vi "Passing Data to a .NET Event Callback.vi"() -> ()   [LabVIEW 2023]
doc: "This vi demonstrates how to use the .NET event callback to fire an event on a value change. This example uses a C# project file to create the event. The constructor from this project is then used to register the event."
uses:
  c:/dev/_r/4/eng/lv-core/lvpostprocessingd/lv_mc_x86_64/dist_i386/examples/Connectivity/Dot NET/EventExample.dll
  EventExample.dll
panel:
  in  "Knob":dbl(knob) scale=0.0..10.0
  in  "Stop":bool
  out "Meter":dbl(knob) scale=0.0..10.0
  # "Overview: Demonstrates how to configure a .NET Event Callback, then pass data to the callback VI when a Value Changed event fires.\nRequirements: Windows\nInstructions:\n1. Run the VI.\n2. Change the Knob value. The value of Meter will be updated based on the knob value sent to the .NET Event Callback VI.\n3. Click Stop to stop the VI."
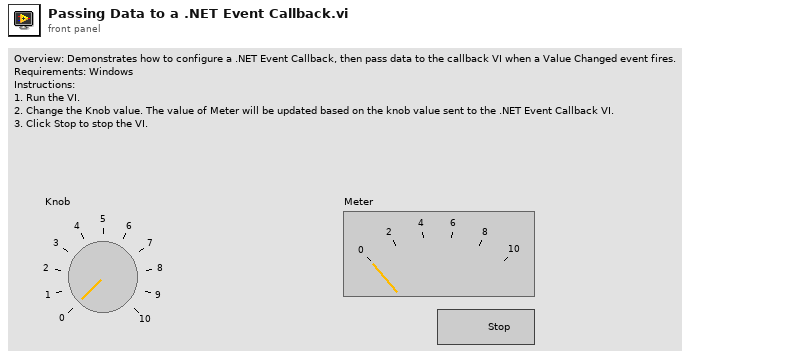
[diagram p1: front panel]
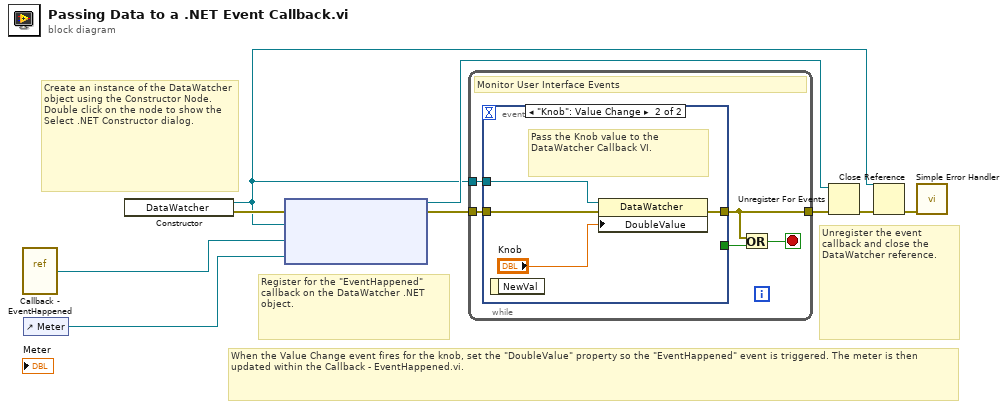
[diagram p0: block diagram]
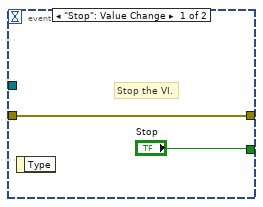
[diagram p2: hidden frame]
diagram:
  # "Create an instance of the DataWatcher object using the Constructor Node. Double click on the node to show the Select .NET Constructor dialog."
  # "When the Value Change event fires for the knob, set the \"DoubleValue\" property so the \"EventHappened\" event is triggered. The meter is then updated within the Callback - EventHappened.vi."
  # "Unregister the event callback and close the DataWatcher reference."
  # "Register for the \"EventHappened\" callback on the DataWatcher .NET object."
  n1 = vi-ref "Callback - EventHappened.vi"() -> ("vi reference"=w1:refnum<vi>)
  n2 = control-ref of="Meter"() -> (w6:refnum<vi>)
  n3 = constructor class="DataWatcher"() -> (reference out=w3:refnum<k24>, error out=w9:errorcluster)  [unwired: 3 in, 1 out]
  n4 = node(w9, w3, w1, w6) -> (w8:refnum<k27>, w4:errorcluster)  [unwired: 1 in]
  n5 = while {
    tunnel: w3 -> [w13]
    tunnel: [w12] -> w5
    tunnel: w4 -> [w10]
    stop <- w11 stop-if-true
    # "Monitor User Interface Events"
    n6 = event shown="[1] \"Knob\": Value Change" {
      selector: _ -> [_ _]
      dyn-events: _ -> [_ _]
      timeout: _ -> [_ _]
      tunnel: ["Stop" _] -> w14
      tunnel: w13 -> [_ w20]
      tunnel: [w15 w19] -> w12
      tunnel: w10 -> [w15 w18]
      event "Stop": Value Change {
        # "Stop the VI."
        n7 = event-data() -> ()  [unwired: 2 out]
      }
      event "Knob": Value Change {
        # "Pass the Knob value to the DataWatcher Callback VI."
        n8 = event-data() -> ()  [unwired: 2 out]
        n9 = property class="DataWatcher"(reference=w20, error in=w18, "DoubleValue"="Knob") -> (error out=w19:errorcluster)  [unwired: 1 out]
      }
    }
    n10 = Or(x=w12, y=w14) -> (x .or. y?=w11:bool)
  }
  n11 = Unregister For Events(event registration refnum=w8, error in=w5) -> (error out=w7:errorcluster)
  n12 = Close Reference(reference=w3, error in (no error)=w7) -> (error out=w2:errorcluster)
  n13 = call <vilib>:"Simple Error Handler.vi"("error in (no error)"=w2) -> ()  [unwired: 4 in, 5 out]
